vi "Read_Endpoint_State.vi"(0 "error in":errorcluster, 2 "Side":T3, 3 "node":string) -> (1 "error out":errorcluster, 4 "Endpoint State":T2)   [LabVIEW 2013]
uses:
  ROS/Code/SubVIs/BaxterSide.ctl
panel:
  out "Orientation":T1
  out "Reply":string
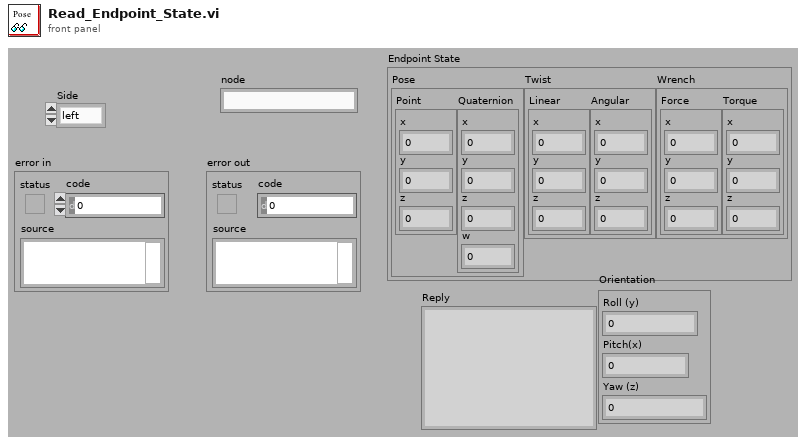
[diagram p1: front panel]
types:
  T1 = cluster{"Roll (y)":dbl, "Pitch(x)":dbl, "Yaw (z)":dbl}
  T2 = cluster{"Pose":cluster{"Point":cluster{"x":dbl, "y":dbl, "z":dbl}, "Quaternion":cluster{"x":dbl, "y":dbl, "z":dbl, "w":dbl}}, "Twist":cluster{"Linear":cluster{"x":dbl, "y":dbl, "z":dbl}, "Angular":cluster{"x":dbl, "y":dbl, "z":dbl}}, "Wrench":cluster{"Force":cluster{"x":dbl, "y":dbl, "z":dbl}, "Torque":cluster{"x":dbl, "y":dbl, "z":dbl}}}
  T3 = typedef "BaxterSide.ctl" = enum16{"left", "right"}
  T4 = typedef "_ROSControl.ctl" = cluster{"topic port":u16, "Node":string, "topic":string, "type":string, "node port":u32, "error ":errorcluster, "Direction":T5, "APIs":string[]}
  T5 = typedef "_ROSDirection.ctl" = enum16{"Node", "Publisher", "Subscriber", "Service Client"}
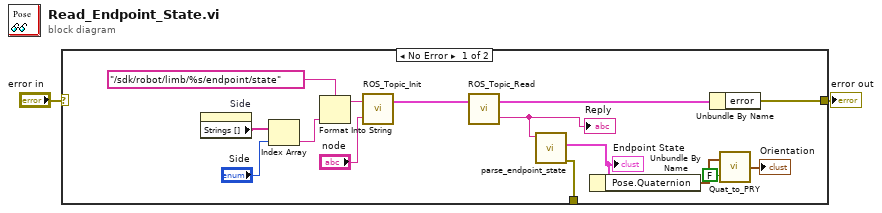
[diagram p0: block diagram]
diagram:
  n1 = case shown="No Error" "error in" {
    selector: "error in" -> [_ w18]
    tunnel: [w17 w18] -> w2
    tunnel: [w7 _] -> _
    frame No Error {
      n2 = property on="Side" class="Enum (strict)"() -> ("Strings []"=w14:string[])  [unwired: 2 in, 2 out]
      n3 = Index Array(array=w14, index="Side") -> (element=w11:string)
      n4 = Format Into String(format string="/sdk/robot/limb/%s/endpoint/state" ("topic"), w11) -> (resulting string=w10:string)  [unwired: 2 in, 1 out]
      n5 = call "ROS_Topic_Init.vi"("node"="node", "topic"=w10) -> ("ROS out"=w15:T4)  [unwired: 1 in]
      n6 = call "ROS_Topic_Read.vi"("ROS in"=w15) -> ("Reply"=w8:string, "ROS out"=w9:T4)  [unwired: 1 in]
      "Reply" <- w8
      n7 = call "parse_endpoint_state.vi"("msg in"=w8) -> ("error out"=w7:errorcluster, "Endpoint State"=w6:T2)  [unwired: 4 in, 1 out]
      "Endpoint State" <- w6
      n8 = Unbundle By Name(w6) -> ("Pose.Quaternion"=w5:cluster{"x":dbl, "y":dbl, "z":dbl, "w":dbl})
      n9 = Unbundle By Name(w9) -> ("error"=w17:errorcluster)
      n10 = call "Quat_to_PRY.vi"("toDegrees? (T)"=FALSE, "Quaternion"=w5) -> ("Orientation"=→"Orientation":T1)
    }
    frame Error {
    }
  }
  "error out" <- w2
